vi "write report.vi"(1 "input":string, 2 "file path (use dialog)":path=path "C:/Users/Garnet/Desktop/New folder/LabView Program/RDUW_v2/test.dat") -> ()   [LabVIEW 2010]
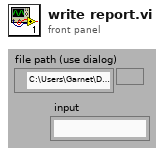
[diagram p1: front panel]
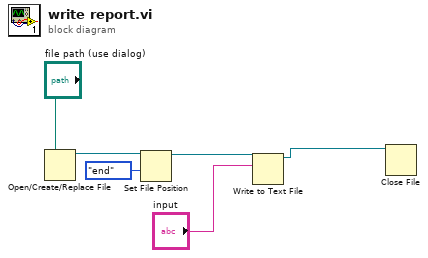
[diagram p0: block diagram]
diagram:
  n1 = Open/Create/Replace File(file path (use dialog)="file path (use dialog)") -> (refnum out=w5:refnum<file>)  [unwired: 5 in, 2 out]
  n2 = Set File Position(refnum=w5, from (0:start)=enum16{"start", "end", "current"}."end") -> (refnum out=w3:refnum<file>)  [unwired: 2 in, 1 out]
  n3 = Write to Text File(file (use dialog)=w3, text="input") -> (refnum out=w1:refnum<file>)  [unwired: 2 in, 2 out]
  n4 = Close File(refnum=w1) -> ()  [unwired: 1 in, 2 out]
